vi "drive.vi"(8 "Speed":dbl=30.0, 9 "Distance (cm)":dbl) -> ()   [LabVIEW 2014, in "Janga.lvrbt"]
uses:
  Janga.lvrbt
  <vilib>/NXT/Block Support/NXT_OutputPort.ctl
  <vilib>/NXT/NXTIO Xnodes/NXTIONodeSubVIs/NXTMotorRunDistance.vi
  <vilib>/NXT/Subs/LVHSConnector.ctl
  <vilib>/NXT/NXTIO Xnodes/AddressXNode/NXTIOAddress.xnode
  <vilib>/NXT/NXTIO Xnodes/NXTIOXNode/NXTIO.xnode
  <vilib>/NXT/LegoClasses/BrickReference/BrickReference.lvclass
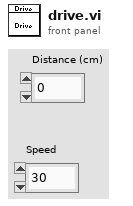
[diagram p1: front panel]
types:
  T1 = typedef "NXT_OutputPort.ctl" = u8
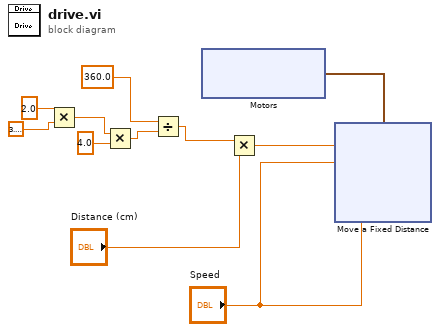
[diagram p0: block diagram]
diagram:
  n1 = Multiply(x=2.0, y=3.141592653589793) -> (x*y=w4:dbl)
  n2 = Multiply(x=w4, y=4.0) -> (x*y=w3:dbl)
  n3 = Divide(x=360.0, y=w3) -> (x/y=w8:dbl)
  n4 = xnode "Motors"() -> ("Motor"=w10:cluster{"Port":T1, "Port":T1})
  n5 = Multiply(x=w8, y="Distance (cm)") -> (x*y=w9:dbl)
  n6 = xnode "Move a Fixed Distance"("Speed 2"="Speed", "Speed 1"="Speed", "Distance 2"=w9, "Distance 1"=w9, "Motors"=w10) -> ()  [unwired: 1 in, 1 out]
